vi "Generator tablic.vi"(1 "Start":dbl=-4.0 format="%#_13g", 2 "Krok":dbl=0.1 format="%#_13g", 3 "End":dbl=4.0 format="%#_13g") -> (0 "Array":dbl[](array[numeric]))   [LabVIEW 2013]
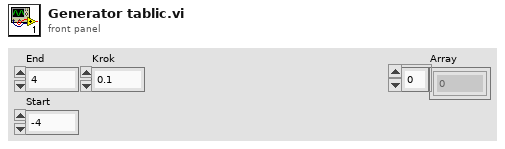
[diagram p1: front panel]
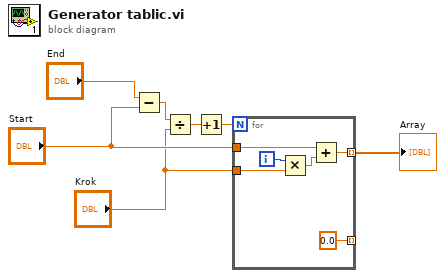
[diagram p0: block diagram]
diagram:
  n1 = Subtract(x="End", y="Start") -> (x-y=w5:dbl)
  n2 = Divide(x=w5, y="Krok") -> (x/y=w3:dbl)
  n3 = Increment(x=w3) -> (x+1=w4:dbl)
  n4 = for {
    N: w4 -> [_]
    tunnel: "Start" -> [w13]
    tunnel: [w12] -> w1 mode=indexing
    tunnel: "Krok" -> [w9]
    tunnel: [0.0] -> _ mode=indexing
    i -> [w11]
    n5 = Multiply(x=w11, y=w9) -> (x*y=w10:dbl)
    n6 = Add(x=w13, y=w10) -> (x+y=w12:dbl)
  }
  "Array" <- w1
